vi "hysModule.vi"(1 "cur_x":dbl=3.0, 2 "cur_p":dbl=4.0, 3 "flag":dbl=1.0) -> (0 "u":dbl)   [LabVIEW 2018]
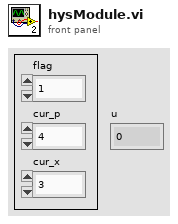
[diagram p1: front panel]
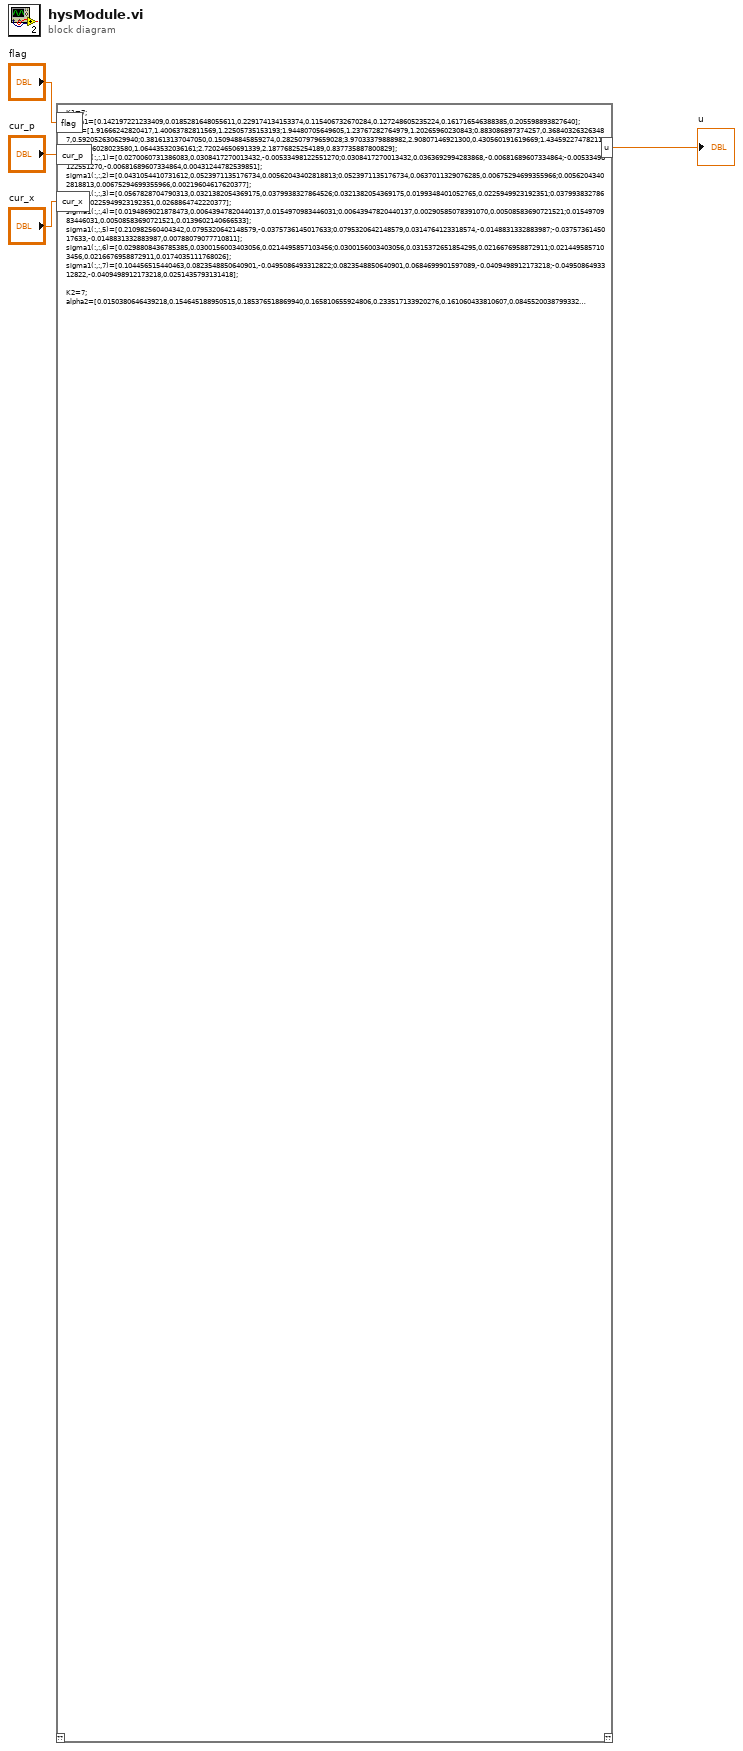
[diagram p0: block diagram]
diagram:
  n1 = script code="K1=7;\nalpha1=[0.142197221233409,0.0185281648055611,0.229174134153374,0.115406732670284,0.127248605235224,0.161716546388385,0.205598893827640];\nmu1=[1.91666242820417,1.40063782811569,1.22505735153193;1.94480705649605,1.23767282764979,1.20265960230843;0.883086897374257,0.368403263263487,0.592052630629940;0.381613137047050,0.150948845859274,0.282507979659028;3.97033379888982,2.90807146921300,0.430560191619669;1.43459227478211,0.830296028023580,1.06443532036161;2.72024650691339,2.18776825254189,0.837735887800829];\nsigma1(:,:,1)=[0.0270060731386083,0.0308417270013432,-0.00533498122551270;0.0308417270013432,0.0363692994283868,-0.00681689607334864;-0.00533498122551270,-0.00681689607334864,0.00431244782539851];\nsigma1(:,:,2)=[0.0431054410731612,0.0523971135176734,0.00562043402818813;0.0523971135176734,0.0637011329076285,0.00675294699355966;0.00562043402818813,0.00675294699355966,0.00219604617620377];\nsigma1(:,:,3)=[0.0567828704790313,0.0321382054369175,0.0379938327864526;0.0321382054369175,0.0199348401052765,0.0225949923192351;0.0379938327864526,0.0225949923192351,0.0268864742220377];\nsigma1(:,:,4)=[0.0194869021878473,0.00643947820440137,0.0154970983446031;0.00643947820440137,0.00290585078391070,0.00508583690721521;0.0154970983446031,0.00508583690721521,0.0139602140666533];\nsigma1(:,:,5)=[0.210982560404342,0.0795320642148579,-0.0375736145017633;0.0795320642148579,0.0314764123318574,-0.0148831332883987;-0.0375736145017633,-0.0148831332883987,0.00788079077710811];\nsigma1(:,:,6)=[0.0298808436785385,0.0300156003403056,0.0214495857103456;0.0300156003403056,0.0315372651854295,0.0216676958872911;0.0214495857103456,0.0216676958872911,0.0174035111768026];\nsigma1(:,:,7)=[0.104456515440463,0.0823548850640901,-0.0495086493312822;0.0823548850640901,0.0684699901597089,-0.0409498912173218;-0.0495086493312822,-0.0409498912173218,0.0251435793131418];\n\nK2=7;\nalpha2=[0.0150380646439218,0.154645188950515,0.185376518869940,0.165810655924806,0.233517133920276,0.161060433810607,0.0845520038799332];\nmu2=[2.53467568049350,2.06119303631039,0.288335690409106;1.09181911876058,0.804457347512283,1.05100334453034;1.76402267850727,1.63352854484466,1.10400100440598;2.59277460960470,2.35230754563918,0.641725527417796;0.535772893387427,0.343647042757828,0.630654202520755;3.82548557544265,2.96918741412406,0.311489218136036;1.63568903999324,1.28367341790766,0.926477638256817];\nsigma2(:,:,1)=[0.239155231823436,0.216936634298939,-0.0377707192000042;0.216936634298939,0.197402357387097,-0.0319500680112039;-0.0377707192000042,-0.0319500680112039,0.0203486494461313];\nsigma2(:,:,2)=[0.0200894985184489,0.0198730506706373,0.0116107689953935;0.0198730506706373,0.0220910776289670,0.0156519501858315;0.0116107689953935,0.0156519501858315,0.0157824242752969];\nsigma2(:,:,3)=[0.0748986308837922,0.0834675810216173,-0.0382579817482540;0.0834675810216173,0.0951841623995514,-0.0412058954666060;-0.0382579817482540,-0.0412058954666060,0.0222433002898511];\nsigma2(:,:,4)=[0.0648843253855970,0.0460543492925619,-0.0277782578844865;0.0460543492925619,0.0371073261804463,-0.0176571681920342;-0.0277782578844865,-0.0176571681920342,0.0137570031916944];\nsigma2(:,:,5)=[0.0407778634782488,0.0253405903153359,0.0245359245362039;0.0253405903153359,0.0161342731459676,0.0158818999383354;0.0245359245362039,0.0158818999383354,0.0168057479453588];\nsigma2(:,:,6)=[0.275334978847715,0.0876972629884982,-0.0499523743155251;0.0876972629884982,0.0291137749415474,-0.0155115714890453;-0.0499523743155251,-0.0155115714890453,0.0109288176943297];\nsigma2(:,:,7)=[0.0350279369873875,0.0329351766579469,-0.0201910439937022;0.0329351766579469,0.0311261676833748,-0.0185861578660877;-0.0201910439937022,-0.0185861578660877,0.0149963734228139];\n\ntmp=[cur_p;cur_x];\nu=1;\n\nif flag==1  \n\n% function dz=H(z,K,alpha,mu,sigma)\nz=tmp;\nK=K1;\nalpha=alpha1;\nmu=mu1;\nsigma=sigma1;\n%===================\ndz=0;\nz=z(:);\nfor k=1:K\n    A(:,:,k)=sigma(3,1:2,k)*inv(sigma(1:2,1:2,k));\n    b(:,k)=mu(k,3)'-A(:,:,k)*mu(k,1:2)';\n    h=0;\n    for j=1:K\n        xx=z;\n        muu=mu(j,1:2);\n        muu=muu(:);\n        sigmaa=sigma(1:2,1:2,j);\n        gau=1/(2*pi*sqrt(det(sigmaa)))*exp(-0.5*(xx-muu)'*inv(sigmaa)*(xx-muu));\n        h=h+alpha(j)*gau;\n    end\n    xx=z;\n    muu=mu(k,1:2);\n    muu=muu(:);\n    sigmaa=sigma(1:2,1:2,k);\n    gau=1/(2*pi*sqrt(det(sigmaa)))*exp(-0.5*(xx-muu)'*inv(sigmaa)*(xx-muu));\n    h=alpha(k)*gau/(h+eps);\n    dz=dz+h*(A(:,:,k)*z+b(:,k));\nend\n\nelseif flag==2\n\n% function dz=H(z,K,alpha,mu,sigma)\nz=tmp;\nK=K2;\nalpha=alpha2;\nmu=mu2;\nsigma=sigma2;\n%===================\ndz=0;\nz=z(:);\nfor k=1:K\n    A(:,:,k)=sigma(3,1:2,k)*inv(sigma(1:2,1:2,k));\n    b(:,k)=mu(k,3)'-A(:,:,k)*mu(k,1:2)';\n    h=0;\n    for j=1:K\n        xx=z;\n        muu=mu(j,1:2);\n        muu=muu(:);\n        sigmaa=sigma(1:2,1:2,j);\n        gau=1/(2*pi*sqrt(det(sigmaa)))*exp(-0.5*(xx-muu)'*inv(sigmaa)*(xx-muu));\n        h=h+alpha(j)*gau;\n    end\n    xx=z;\n    muu=mu(k,1:2);\n    muu=muu(:);\n    sigmaa=sigma(1:2,1:2,k);\n    gau=1/(2*pi*sqrt(det(sigmaa)))*exp(-0.5*(xx-muu)'*inv(sigmaa)*(xx-muu));\n    h=alpha(k)*gau/(h+eps);\n    dz=dz+h*(A(:,:,k)*z+b(:,k));\nend\n\nend\nu=dz;" ("脚本节点")("flag"="flag", "cur_x"="cur_x", "cur_p"="cur_p") -> ("u"=→"u":dbl)  [unwired: 1 in, 1 out]
